vi "Get Path.vi"(8 "error in (no error)":errorcluster, 11 "File Response in":refnum<class "File Response.lvclass">) -> (0 "error out":errorcluster, 2 "Path":path, 3 "File Response out":refnum<class "File Response.lvclass">)   [LabVIEW 2020, in "HTTP Server.lvlib" / "File Response.lvclass"]
uses:
  File Response.lvclass
  File Response.lvclass/File Response.ctl
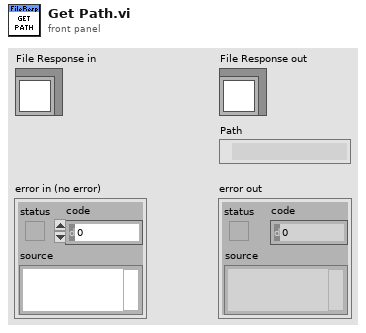
[diagram p1: front panel]
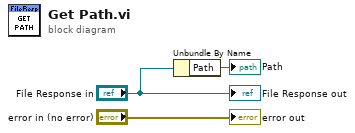
[diagram p0: block diagram]
diagram:
  n1 = Unbundle By Name("File Response in") -> ("Path"=→"Path":path)
  "error out" <- "error in (no error)"
  "File Response out" <- "File Response in"
